vi "NXT P string B.vi"(0 "string":string="32-9123456", 1 "error in":errorcluster) -> (2 "Desired Velocity":i16, 3 "Local Heading":i16, 4 "Mode":i16, 5 "error out":errorcluster)   [LabVIEW 2012, in "ENGR3390 Tug Boat.lvrbt"]
doc: "This VI parses the values of a string passed as a \"P\" from the PC."
uses:
  ENGR3390 Tug Boat.lvrbt
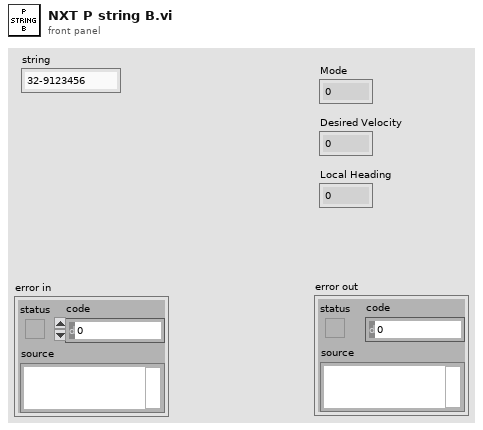
[diagram p1: front panel]
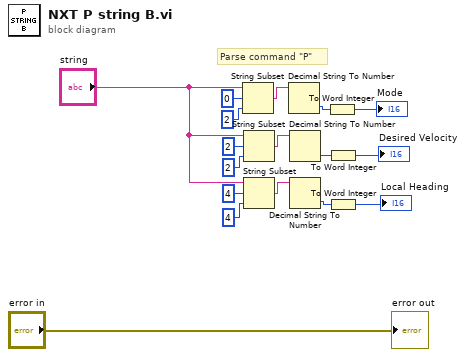
[diagram p0: block diagram]
diagram:
  # "Parse command \"P\""
  n1 = String Subset(string="string", offset (0)=0, length (rest)=2 ("length (rest)")) -> (substring=w17:string)
  n2 = String Subset(string="string", offset (0)=2, length (rest)=2 ("length (rest)")) -> (substring=w11:string)
  n3 = String Subset(string="string", offset (0)=4, length (rest)=4 ("length (rest)")) -> (substring=w7:string)
  n4 = Decimal String To Number(string=w17) -> (number=w14:i32)  [unwired: 2 in, 1 out]
  n5 = Decimal String To Number(string=w11) -> (number=w10:i32)  [unwired: 2 in, 1 out]
  n6 = Decimal String To Number(string=w7) -> (number=w9:i32)  [unwired: 2 in, 1 out]
  n7 = To Word Integer(number=w14) -> (16bit integer=→"Mode":i16)
  n8 = To Word Integer(number=w10) -> (16bit integer=→"Desired Velocity":i16)
  n9 = To Word Integer(number=w9) -> (16bit integer=→"Local Heading":i16)
  "error out" <- "error in"
